vi "configREF.vi"(7 "address":string, 8 "error in (no error)":errorcluster, 11 "Channels: Lockin in":T1 {"REF phi (deg)" format="%#_3g"}) -> (0 "error out":errorcluster, 3 "Channels: Lockin out":T1 {"REF phi (deg)" format="%#_3g"})   [LabVIEW 2016]
doc: "API to configure the REF.\n\nIf address=\"\", this API reads from localhost\nIf address is remote lockin, you need to add this computer to allowed whitelist on the lockin computer you are trying to access."
uses:
  Typedefs/REF-cluster.ctl
  Typedefs/REF_f-array.ctl
  Typedefs/REF_phi-array.ctl
  SMOs/RemoteControl/Typedefs/Remote-SMO-Commands-Enum.ctl
  <vilib>/addons/_JKI.lib/Serialization/JSON/JKI JSON Serialization.lvlib
  SMOs/RemoteControl/RemoteControl.lvclass
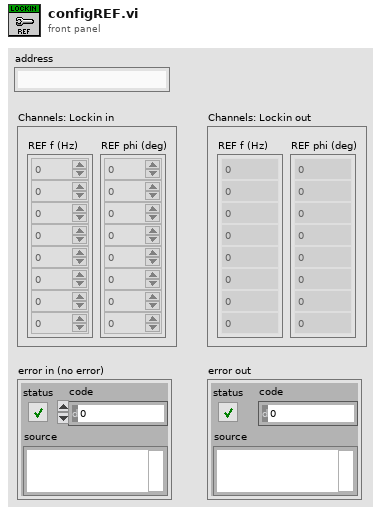
[diagram p1: front panel]
types:
  T1 = typedef "REF-cluster.ctl" = cluster{"REF f (Hz)":T2, "REF phi (deg)":T3}
  T2 = typedef "REF_f-array.ctl" = dbl[]
  T3 = typedef "REF_phi-array.ctl" = dbl[]
  T4 = typedef "RemoteControl.lvclass/Remote-SMO-Commands-Enum.ctl" = enum16{"configAO", "configREF", "configIVmode", "configRemote", "configReset", "assertTrigger", "getAO", "getAI", "getResults", "getTrigger", "getIVmode", "getAOconfig", "getREFconfig", "ACK", "UNK", "CLOSE"}
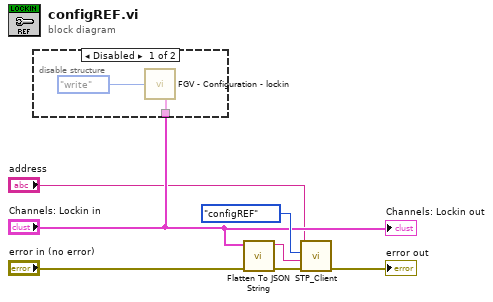
[diagram p0: block diagram]
diagram:
  n1 = disable-structure shown="Disabled" {
    disable-tunnel: "Channels: Lockin in" -> [w8 _]
    frame Disabled {
      n2 = call "FGV - Configuration - lockin.vi"("Function"=enum16{"write", "read"}."write", "Channels: Lockin"=w8) -> ()  [unwired: 4 in, 2 out]
    }
    frame Enabled {
    }
  }
  n3 = call <vilib>:"Flatten To JSON String.vi"("error in (no error)"="error in (no error)", "Variant"="Channels: Lockin in") -> ("error out"=w7:errorcluster, "JSON String"=w6:string)  [unwired: 8 in]
  n4 = call "STP_Client.vi"("error in (no error)"=w7, "data to send"=w6, "Command"=Remote-SMO-Commands-Enum."configREF", "address"="address") -> ("error out"=→"error out":errorcluster)  [unwired: 6 in, 1 out]
  "Channels: Lockin out" <- "Channels: Lockin in"
